vi "GoTo.vi"(3 "error in (no error)":errorcluster, 4 "Wavelength":u16, 5 "VISA resource name":refnum<visa-resource-name>) -> (0 "error out":errorcluster, 1 "Command not accepted":bool, 2 "VISA resource name out":refnum<visa-resource-name>)   [LabVIEW 2017, in "Spectral Products CM110.lvlib"]
uses:
  Spectral Products CM110.lvlib
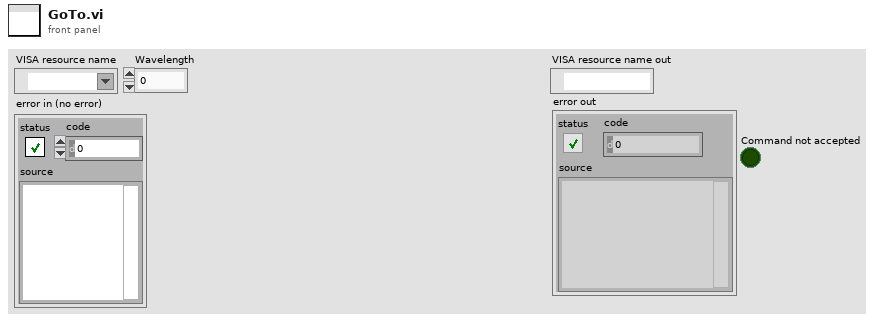
[diagram p1: front panel]
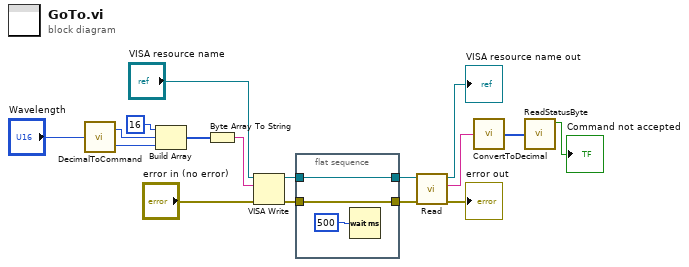
[diagram p0: block diagram]
diagram:
  n1 = call "DecimalToCommand.vi"("Decimal"="Wavelength") -> ("HiByte"=w8:u8, "LoByte"=w7:u8)  [unwired: 4 in]
  n2 = Build Array(u8 16, w8, w7) -> (w6:u8[])
  n3 = Byte Array To String(unsigned byte array=w6) -> (string=w5:string)
  n4 = VISA Write(VISA resource name="VISA resource name", write buffer=w5, error in (no error)="error in (no error)") -> (VISA resource name out=w3:refnum<visa-resource-name>, error out=w2:errorcluster)  [unwired: 1 out]
  n5 = flat-sequence {
    tunnel: [w20] -> w4
    tunnel: w3 -> [w20]
    tunnel: w2 -> [w19]
    tunnel: [w19] -> w1
    frame #0 {
      n6 = Wait (ms)(milliseconds to wait=u32 500) -> ()  [unwired: 1 out]
    }
  }
  n7 = call "Read.vi"("error in (no error)"=w1, "VISA Refnum in"=w4) -> ("error out"=→"error out":errorcluster, "read buffer"=w13:string, "VISA Refnum out"=→"VISA resource name out":refnum<visa-resource-name>)  [unwired: 6 in, 1 out]
  n8 = call "ConvertToDecimal.vi"("read buffer"=w13) -> ("unsigned byte array"=w12:u8[])
  n9 = call "ReadStatusByte.vi"("unsigned byte array"=w12) -> ("Command not accepted"=→"Command not accepted":bool)  [unwired: 4 in, 5 out]
